vi "Array of Variants to JSON Array.vi"(5 "enable LabVIEW extensions? (T)":bool=TRUE, 6 "Pretty Print?":bool, 9 "error in (no error)":errorcluster, 11 "Array of Variants":variant[](array[variant])) -> (1 "error out":errorcluster, 3 "<JSON>":string)   [LabVIEW 2015, in "JSONtext.lvlib"]
doc: "Flatten an Array of Variants into a JSON Array. \n\nStrings or Arrays of strings marked with a leading \"<JSON>\" tag in their name (including inside clusters) are treated as already being valid JSON. Strings not marked as <JSON> are quoted and escaped as a JSON String."
uses:
  JSONtext.lvlib
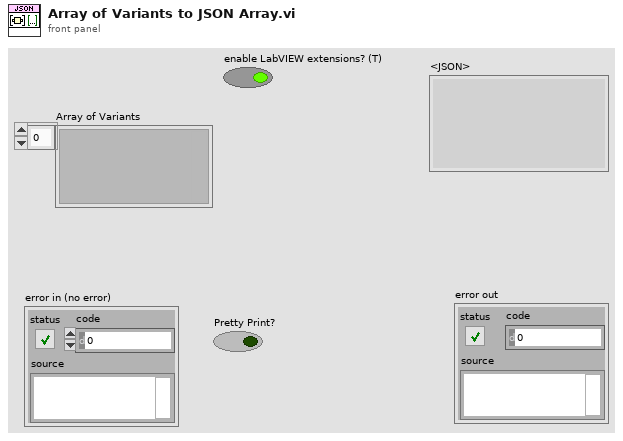
[diagram p1: front panel]
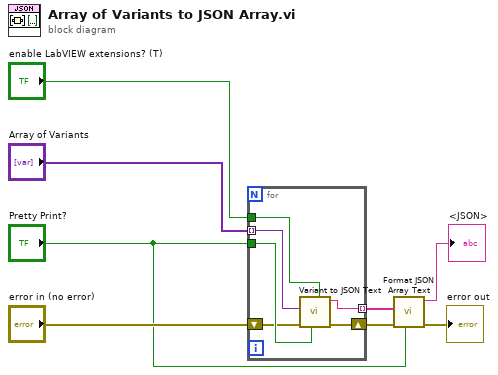
[diagram p0: block diagram]
diagram:
  n1 = for {
    tunnel: "Array of Variants" -> [w14] mode=indexing
    tunnel: "Pretty Print?" -> [w13]
    tunnel: [w9] -> w3 mode=indexing
    shift-right: [w12] -> w6
    shift-left: "error in (no error)" -> [w11]
    tunnel: "enable LabVIEW extensions? (T)" -> [w10]
    n2 = call "Variant to JSON Text.vi"("enable LabVIEW extensions? (T)"=w10, "Pretty Print?"=w13, "error in (no error)"=w11, "Variant"=w14) -> ("error out"=w12:errorcluster, "<JSON>"=w9:string)  [unwired: 5 in, 1 out]
  }
  n3 = call "Format JSON Array Text.vi"("Pretty Print?"="Pretty Print?", "error in (no error)"=w6, "Array of JSON Text"=w3) -> ("error out"=→"error out":errorcluster, "<JSON>"=→"<JSON>":string)  [unwired: 7 in]
